vi "Open Excel Report.vi"(8 "error in":errorcluster, 10 "Filename":string, 11 "Base Path":path) -> (0 "error out":errorcluster)   [LabVIEW 2012]
panel:
  in  "Excel._Application":refnum<k7>
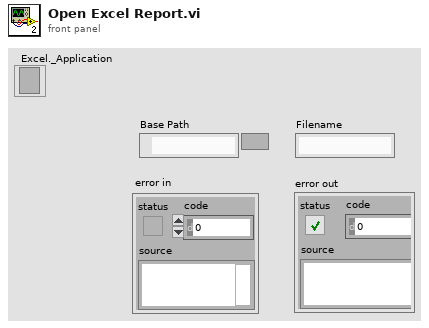
[diagram p1: front panel]
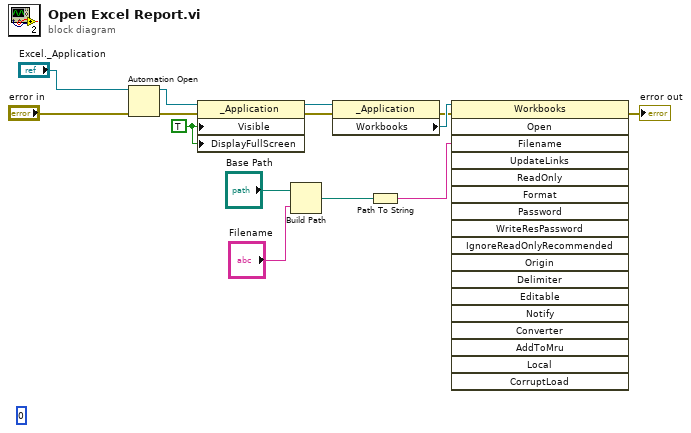
[diagram p0: block diagram]
diagram:
  (unwired) 0
  w2 = TRUE ("Visible Boolean")
  n1 = Automation Open(error in (no error)="error in", Automation Refnum="Excel._Application") -> (Automation Refnum=w13:refnum<k7>, error out=w14:errorcluster)  [unwired: 2 in]
  n2 = property class="_Application"(reference=w13, error in=w14, "Visible"=w2, "DisplayFullScreen"=w2) -> (reference out=w9:refnum<k7>, error out=w8:errorcluster)
  n3 = Build Path(base path="Base Path", name or relative path="Filename") -> (appended path=w5:path)
  n4 = property class="_Application"(reference=w9, error in=w8) -> (error out=w10:errorcluster, "Workbooks"=w11:refnum<k7>)  [unwired: 1 out]
  n5 = Path To String(path=w5) -> (string=w4:string)
  n6 = invoke class="Workbooks" method="Open"(reference=w11, error in=w10, "Filename"=w4) -> (error out=→"error out":errorcluster)  [unwired: 15 in, 17 out]
